vi "ConvertFromDynamicDataType.vi"() -> ()   [LabVIEW 2019]
uses:
  <vilib>/measure/NI_MABase.lvlib
panel:
  out "Distance":dbl[unit]
  in  "Time":dbl[unit]
  in  "Speed":dbl[unit]
  in  "String":string
  out "rest of the binary string":string
  out "data string":string
  in  "Numeric value":dbl
  in  "Stop Wave Genrations":bool
  out "appended array":waveform(dbl)[][](array[waveform])
  in  "phase":dbl format="%.2p"
  in  "amplitude":dbl=1.0 format="%0.2p"
  in  "frequency":dbl=10.0 format="%0.2p"
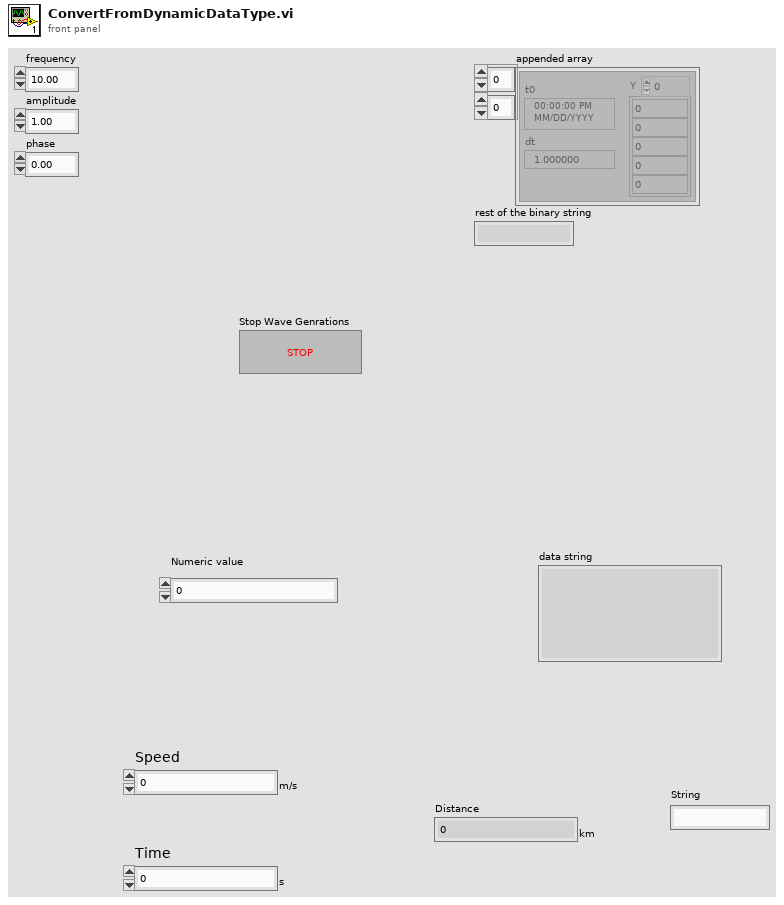
[diagram p1: front panel]
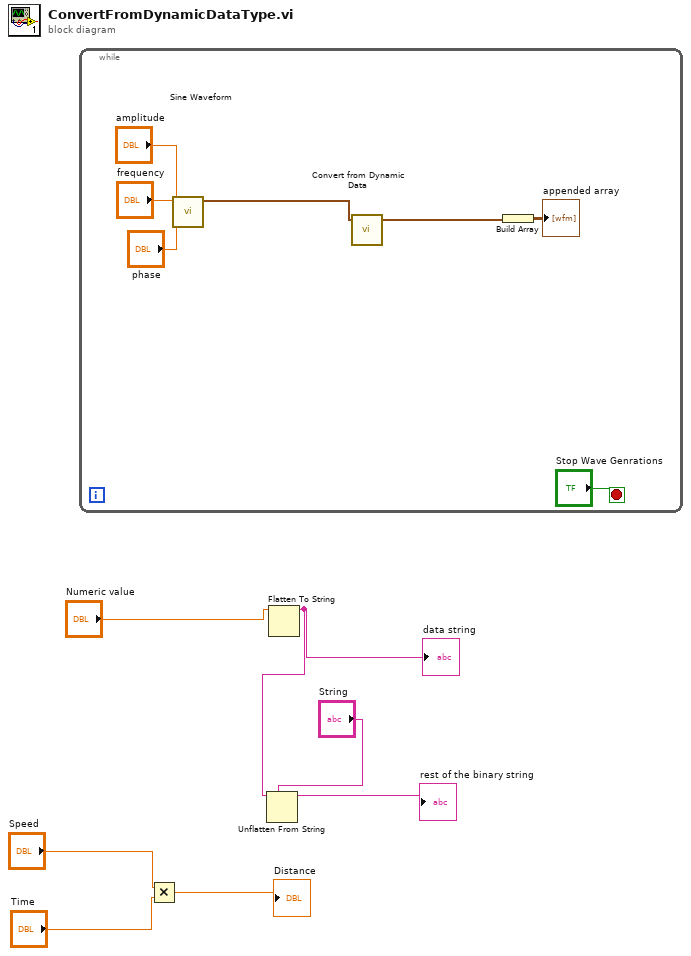
[diagram p0: block diagram]
diagram:
  n1 = while {
    stop <- "Stop Wave Genrations" stop-if-true
    n2 = call <vilib>:"Sine Waveform.vi"("phase"="phase", "amplitude"="amplitude", "frequency"="frequency") -> ("signal out"=w10:waveform(dbl))  [unwired: 7 in, 1 out]
    n3 = call "Convert from Dynamic Data"("Dynamic Data Type"=w10) -> ("Array of Waveform"=w14:waveform(dbl)[])  [unwired: 3 in]
    n4 = Build Array "Build Array"(w14) -> (→"appended array":waveform(dbl)[][])
  }
  n5 = Multiply(x="Speed", y="Time") -> (x*y=→"Distance":dbl[unit])
  n6 = Flatten To String(anything="Numeric value") -> (data string=w6:string)  [unwired: 3 in, 2 out]
  "data string" <- w6
  n7 = Unflatten From String(type="String", binary string=w6) -> (rest of the binary string=→"rest of the binary string":string)  [unwired: 3 in, 2 out]
